vi "Is Channel Enabled.vi"(8 "error in (no error)":errorcluster, 10 "Channel (0: Channel 1)":u16(ring) items=["Channel 1", "Channel 2", "Channel 3", "Channel 4", "Math", "Reference 1", "Reference 2", "Reference 3", "Reference 4", "Normal", "Average", "Amplitude", "Frequency", "Minimum Peak Hold", "Maximum Peak Hold", "Phase", "Digital Channel 0", "Digital Channel 1", "Digital Channel 2", "Digital Channel 3", "Digital Channel 4", "Digital Channel 5", "Digital Channel 6", "Digital Channel 7", "Digital Channel 8", "Digital Channel 9", "Digital Channel 10", "Digital Channel 11", "Digital Channel 12", "Digital Channel 13", "Digital Channel 14", "Digital Channel 15"], 11 "VISA resource name":refnum<visa-resource-name>) -> (0 "error out":errorcluster, 2 "Enabled":bool, 3 "VISA resource name out":refnum<visa-resource-name>)   [LabVIEW 2016, in "Tektronix DPO MSO 2000 4000 Series.lvlib"]
doc: "Queries whether the specified input channel is enabled to acquire a waveform from the oscilloscope."
uses:
  Tektronix DPO MSO 2000 4000 Series.lvlib
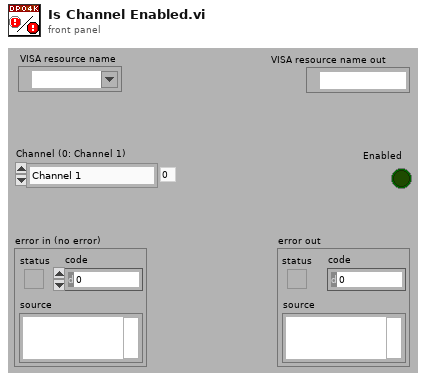
[diagram p1: front panel]
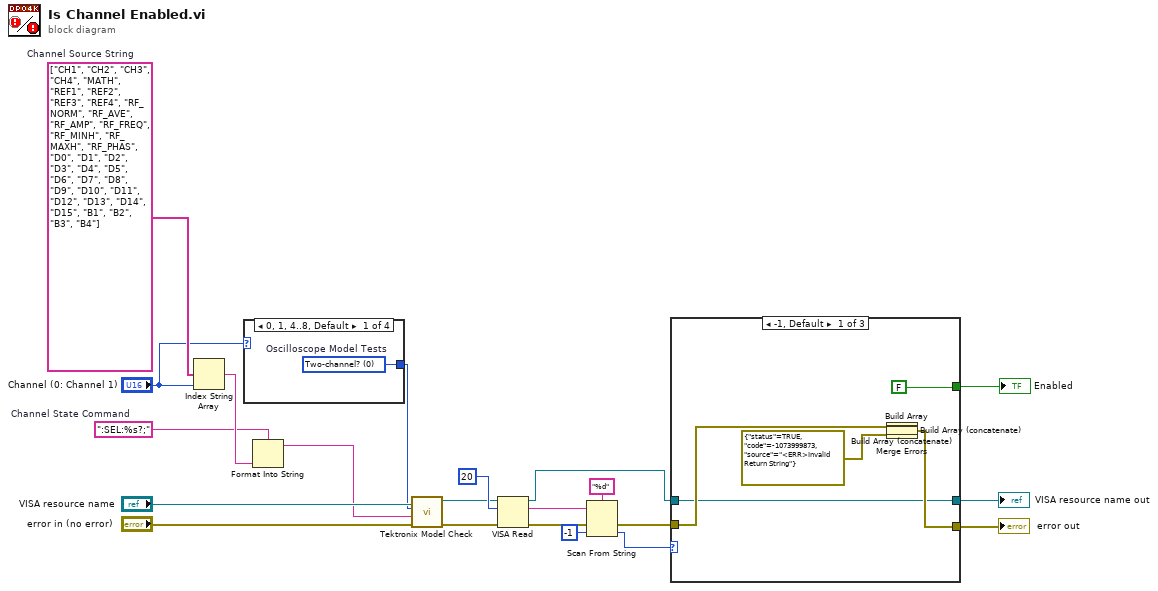
[diagram p0: block diagram]
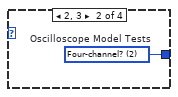
[diagram p2: hidden frame]
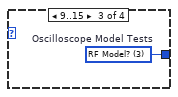
[diagram p3: hidden frame]
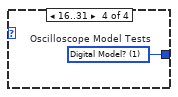
[diagram p4: hidden frame]
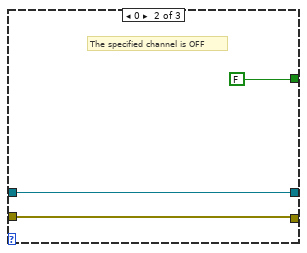
[diagram p5: hidden frame]
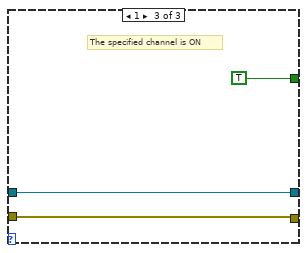
[diagram p6: hidden frame]
diagram:
  w10 = ":SEL:%s?;"  # Channel State Command
  w9 = string[] ["CH1", "CH2", "CH3", "CH4", "MATH", "REF1", "REF2", "REF3", "REF4", "RF_NORM", "RF_AVE", "RF_AMP", "RF_FREQ", "RF_MINH", "RF_MAXH", "RF_PHAS", "D0", "D1", "D2", "D3", "D4", "D5", "D6", "D7", "D8", "D9", "D10", "D11", "D12", "D13", "D14", "D15", "B1", "B2", "B3", "B4"]  # Channel Source String
  n1 = Index String Array(1:"Channel (0: Channel 1)", 2:w9) -> (0:w11:string)  [unwired: 1 in]
  n2 = case shown="0, 1, 4..8, Default" "Channel (0: Channel 1)" {
    tunnel: [w22 w23 w24 w25] -> w4
    frame 0, 1, 4..8, Default {
      w22 = u16 0 items=["Two-channel?", "Digital Model?", "Four-channel?", "RF Model?"]  # Oscilloscope Model Tests
    }
    frame 2, 3 {
      w23 = u16 2 items=["Two-channel?", "Digital Model?", "Four-channel?", "RF Model?"]  # Oscilloscope Model Tests
    }
    frame 9..15 {
      w24 = u16 3 items=["Two-channel?", "Digital Model?", "Four-channel?", "RF Model?"]  # Oscilloscope Model Tests
    }
    frame 16..31 {
      w25 = u16 1 items=["Two-channel?", "Digital Model?", "Four-channel?", "RF Model?"]  # Oscilloscope Model Tests
    }
  }
  n3 = Format Into String(format string=w10, w11) -> (resulting string=w1:string)  [unwired: 2 in, 1 out]
  n4 = call "Tektronix Model Check.vi"("error in (no error)"="error in (no error)", "Command String"=w1, "Oscilloscope Model Tests (3: RF Model?)"=w4, "VISA resource name"="VISA resource name") -> ("error out"=w2:errorcluster, "VISA resource name out"=w3:refnum<visa-resource-name>)  [unwired: 6 in]
  n5 = VISA Read(VISA resource name=w3, byte count=u32 20, error in (no error)=w2) -> (VISA resource name out=w19:refnum<visa-resource-name>, read buffer=w15:string, error out=w16:errorcluster)  [unwired: 1 out]
  n6 = Scan From String(format string="%d", input string=w15, error in=w16, default 1=-1 ("default value 1")) -> (error out=w18:errorcluster, output 1=w21:i32)  [unwired: 1 in, 2 out]
  n7 = case shown="-1, Default" w21 {
    tunnel: w19 -> [w30 w36 w39]
    tunnel: w18 -> [w32 w35 w37]
    tunnel: [w31 w35 w37] -> w14
    tunnel: [w30 w36 w39] -> w13
    tunnel: [FALSE FALSE TRUE] -> w8
    frame -1, Default {
      n8 = Build Array(w32, errorcluster {"status"=TRUE, "code"=-1073999873, "source"="<ERR>Invalid Return String"} ("error out")) -> (w28:errorcluster[])
      n9 = Build Array (concatenate)(w28) -> (w27:errorcluster[])
      n10 = Build Array (concatenate)(w27) -> (w26:errorcluster[])
      n11 = Merge Errors(w26) -> (w31:errorcluster)
    }
    frame 0 {
      # "The specified channel is OFF"
    }
    frame 1 {
      # "The specified channel is ON"
    }
  }
  "error out" <- w14
  "VISA resource name out" <- w13
  "Enabled" <- w8
